vi "Read Write Config.vi"(0 "Config File":path, 2 "Read?":bool, 7 "Cluster In":T2, 11 "Error In":errorcluster) -> (8 "Cluster Out":T2, 15 "Error Out":errorcluster)   [LabVIEW 2013]
uses:
  TypeDef/StandConfigCluster.ctl
  <vilib>/Utility/config.llb/Write Key (String).vi
  <vilib>/Utility/config.llb/Write Key (Double).vi
  <vilib>/Utility/config.llb/Write Key (I32).vi
  <vilib>/Utility/config.llb/Read Key (String).vi
  <vilib>/Utility/config.llb/Read Key (Double).vi
  <vilib>/Utility/config.llb/Read Key (I32).vi
  <vilib>/Utility/config.llb/NI_LVConfig.lvlib
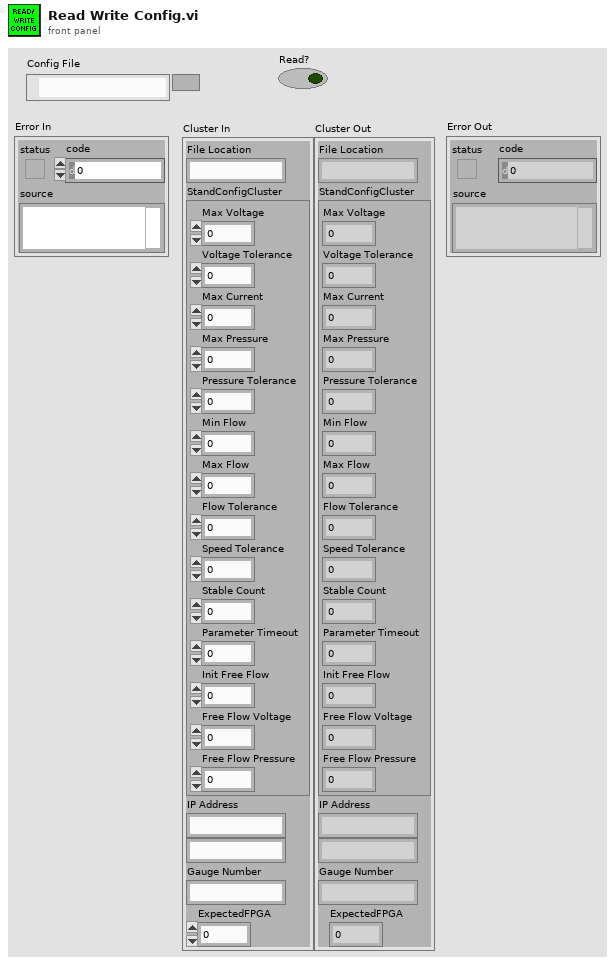
[diagram p1: front panel]
types:
  T1 = typedef "StandConfigCluster.ctl" = cluster{"Max Voltage":dbl, "Voltage Tolerance":dbl, "Max Current":dbl, "Max Pressure":dbl, "Pressure Tolerance":dbl, "Min Flow":dbl, "Max Flow":dbl, "Flow Tolerance":dbl, "Speed Tolerance":dbl, "Stable Count":dbl, "Parameter Timeout":dbl, "Init Free Flow":dbl, "Free Flow Voltage":dbl, "Free Flow Pressure":dbl}
  T2 = cluster{"File Location":string, "StandConfigCluster":T1, "IP Address":string, string, "Gauge Number":string, "ExpectedFPGA":i32}
  T3 = enum16{"open", "replace", "create", "open or create", "replace or create", "replace or create with confirmation"}
  T4 = typedef "NI_LVConfig.lvlib/Config Data RefNum.ctl" = refnum<k1>
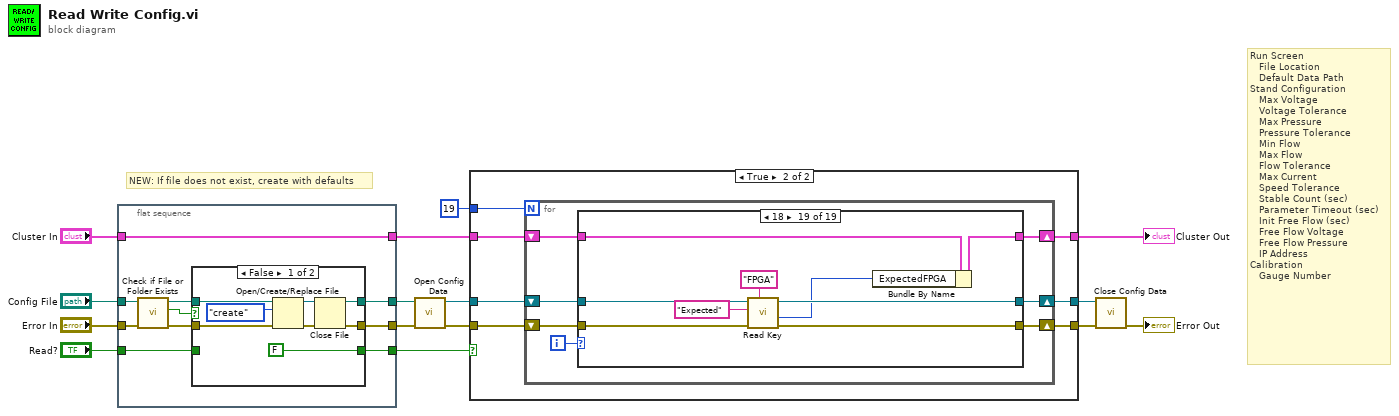
[diagram p0: block diagram]
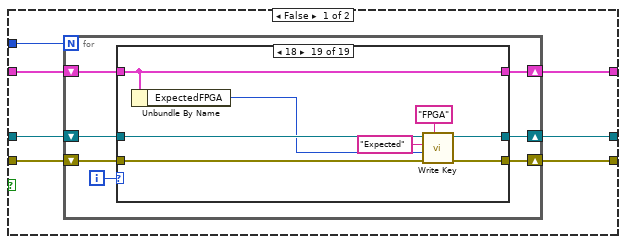
[diagram p3: hidden frame]
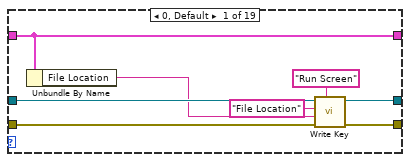
[diagram p4: hidden frame]
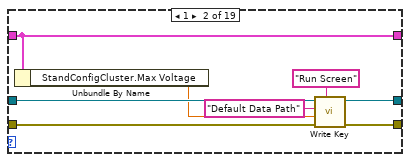
[diagram p5: hidden frame]
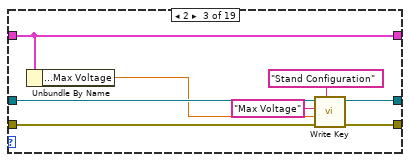
[diagram p6: hidden frame]
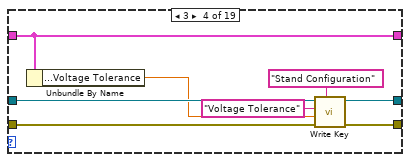
[diagram p7: hidden frame]
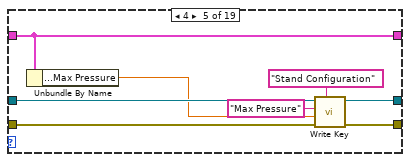
[diagram p8: hidden frame]
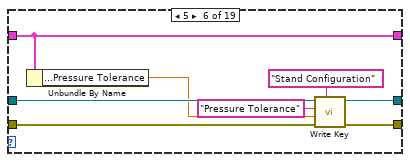
[diagram p9: hidden frame]
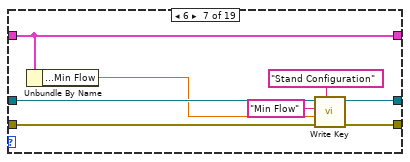
[diagram p10: hidden frame]
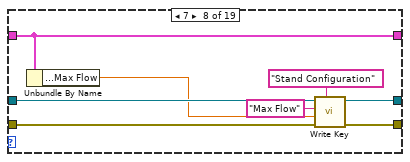
[diagram p11: hidden frame]
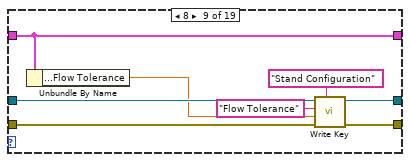
[diagram p12: hidden frame]
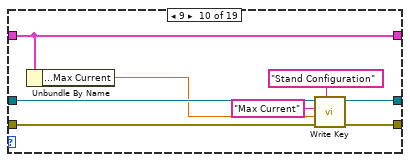
[diagram p13: hidden frame]
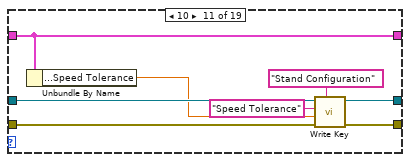
[diagram p14: hidden frame]
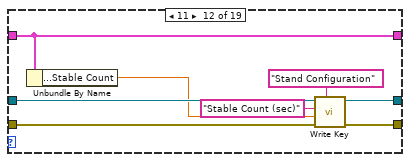
[diagram p15: hidden frame]
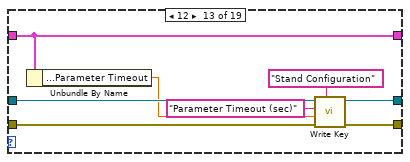
[diagram p16: hidden frame]
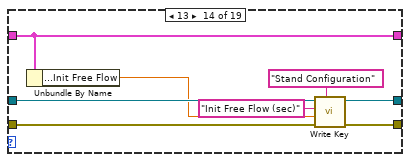
[diagram p17: hidden frame]
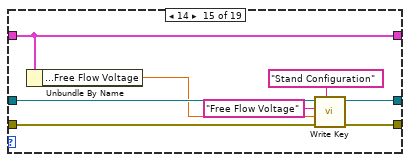
[diagram p18: hidden frame]
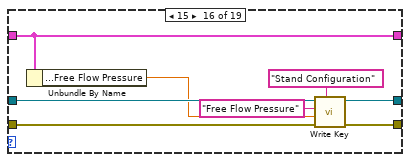
[diagram p19: hidden frame]
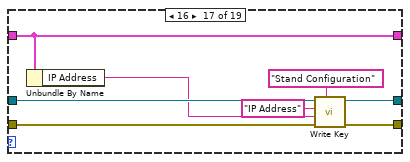
[diagram p20: hidden frame]
diagram:
  # "NEW: If file does not exist, create with defaults"
  # "Run Screen\n   File Location\n   Default Data Path\nStand Configuration\n   Max Voltage\n   Voltage Tolerance\n   Max Pressure\n   Pressure Tolerance\n   Min Flow\n   Max Flow\n   Flow Tolerance\n   Max Current\n   Speed Tolerance\n   Stable Count (sec)\n   Parameter Timeout (sec)\n   Init Free Flow (sec)\n   Free Flow Voltage\n   Free Flow Pressure\n   IP Address\nCalibration\n   Gauge Number"
  n1 = flat-sequence {
    tunnel: "Cluster In" -> [w25]
    tunnel: "Config File" -> [w24]
    tunnel: "Error In" -> [w23]
    tunnel: "Read?" -> [w17]
    tunnel: [w25] -> w7
    tunnel: [w19] -> w6
    tunnel: [w18] -> w5
    tunnel: [w16] -> w4
    frame #0 {
      n2 = call <vilib>:"Check if File or Folder Exists.vi"("error in (no error)"=w23, "path"=w24) -> ("error out"=w21:errorcluster, "file or folder exists?"=w22:bool, "dup path"=w20:path)  [unwired: 7 in]
      n3 = case shown="False" w22 {
        tunnel: [w28 w36] -> w18
        tunnel: w21 -> [w31 w36]
        tunnel: [w27 w35] -> w19
        tunnel: w20 -> [w32 w35]
        tunnel: [FALSE w34] -> w16
        tunnel: w17 -> [_ w34]
        frame False {
          n4 = Open/Create/Replace File(file path (use dialog)=w32, error in=w31, operation (0:open)=T3."create") -> (refnum out=w26:refnum<file>, error out=w29:errorcluster)  [unwired: 3 in, 1 out]
          n5 = Close File(refnum=w26, error in=w29) -> (path=w27:path, error out=w28:errorcluster)
        }
        frame True {
        }
      }
    }
  }
  n6 = call <vilib>:"Open Config Data.vi"("error in (no error)"=w5, "configuration file path"=w6) -> ("error out"=w14:errorcluster, "refnum"=w15:T4)  [unwired: 7 in, 1 out]
  n7 = case shown="True" w4 {
    tunnel: w15 -> [w43 w209]
    tunnel: w14 -> [w42 w208]
    tunnel: [w41 w207] -> w13
    tunnel: [w40 w206] -> w12
    tunnel: w7 -> [w39 w205]
    tunnel: [w38 w204] -> w1
    tunnel: 19 -> [w37 w203]
    frame False {
      n8 = for {
        N: w37 -> [_]
        shift-right: [w48] -> w41
        shift-left: w43 -> [w50]
        shift-right: [w47] -> w40
        shift-left: w42 -> [w49]
        shift-right: [w44] -> w38
        shift-left: w39 -> [w45]
        i -> [w46]
        n9 = case shown="18" w46 {
          tunnel: w50 -> [w58 w66 w74 w82 w90 w98 w106 w114 w122 w130 w138 w146 w154 w162 w170 w178 w186 w194 w202]
          tunnel: w49 -> [w57 w65 w73 w81 w89 w97 w105 w113 w121 w129 w137 w145 w153 w161 w169 w177 w185 w193 w201]
          tunnel: [w56 w64 w72 w80 w88 w96 w104 w112 w120 w128 w136 w144 w152 w160 w168 w176 w184 w192 w200] -> w48
          tunnel: [w55 w63 w71 w79 w87 w95 w103 w111 w119 w127 w135 w143 w151 w159 w167 w175 w183 w191 w199] -> w47
          tunnel: w45 -> [w52 w60 w68 w76 w84 w92 w100 w108 w116 w124 w132 w140 w148 w156 w164 w172 w180 w189 w197]
          tunnel: [w52 w60 w68 w76 w84 w92 w100 w108 w116 w124 w132 w140 w148 w156 w164 w172 w180 w189 w197] -> w44
          frame 0, Default {
            n10 = Unbundle By Name(w52) -> ("File Location"=w51:string)
            n11 = call-poly <vilib>:"Write Key.vi"("section"="Run Screen", "error in (no error)"=w57, "value"=w51, "key"="File Location", "refnum"=w58) -> ("error out"=w55:errorcluster, "refnum out"=w56:T4)  [unwired: 4 in, 1 out]
          }
          frame 1 {
            n12 = Unbundle By Name(w60) -> ("StandConfigCluster.Max Voltage"=w59:dbl)
            n13 = call-poly <vilib>:"Write Key.vi"("section"="Run Screen", "error in (no error)"=w65, "value"=w59, "key"="Default Data Path", "refnum"=w66) -> ("error out"=w63:errorcluster, "refnum out"=w64:T4)  [unwired: 4 in, 1 out]
          }
          frame 2 {
            n14 = Unbundle By Name(w68) -> ("StandConfigCluster.Max Voltage"=w67:dbl)
            n15 = call-poly <vilib>:"Write Key.vi"("section"="Stand Configuration", "error in (no error)"=w73, "value"=w67, "key"="Max Voltage", "refnum"=w74) -> ("error out"=w71:errorcluster, "refnum out"=w72:T4)  [unwired: 4 in, 1 out]
          }
          frame 3 {
            n16 = Unbundle By Name(w76) -> ("StandConfigCluster.Voltage Tolerance"=w75:dbl)
            n17 = call-poly <vilib>:"Write Key.vi"("section"="Stand Configuration", "error in (no error)"=w81, "value"=w75, "key"="Voltage Tolerance", "refnum"=w82) -> ("error out"=w79:errorcluster, "refnum out"=w80:T4)  [unwired: 4 in, 1 out]
          }
          frame 4 {
            n18 = Unbundle By Name(w84) -> ("StandConfigCluster.Max Pressure"=w83:dbl)
            n19 = call-poly <vilib>:"Write Key.vi"("section"="Stand Configuration", "error in (no error)"=w89, "value"=w83, "key"="Max Pressure", "refnum"=w90) -> ("error out"=w87:errorcluster, "refnum out"=w88:T4)  [unwired: 4 in, 1 out]
          }
          frame 5 {
            n20 = Unbundle By Name(w92) -> ("StandConfigCluster.Pressure Tolerance"=w91:dbl)
            n21 = call-poly <vilib>:"Write Key.vi"("section"="Stand Configuration", "error in (no error)"=w97, "value"=w91, "key"="Pressure Tolerance", "refnum"=w98) -> ("error out"=w95:errorcluster, "refnum out"=w96:T4)  [unwired: 4 in, 1 out]
          }
          frame 6 {
            n22 = Unbundle By Name(w100) -> ("StandConfigCluster.Min Flow"=w99:dbl)
            n23 = call-poly <vilib>:"Write Key.vi"("section"="Stand Configuration", "error in (no error)"=w105, "value"=w99, "key"="Min Flow", "refnum"=w106) -> ("error out"=w103:errorcluster, "refnum out"=w104:T4)  [unwired: 4 in, 1 out]
          }
          frame 7 {
            n24 = Unbundle By Name(w108) -> ("StandConfigCluster.Max Flow"=w107:dbl)
            n25 = call-poly <vilib>:"Write Key.vi"("section"="Stand Configuration", "error in (no error)"=w113, "value"=w107, "key"="Max Flow", "refnum"=w114) -> ("error out"=w111:errorcluster, "refnum out"=w112:T4)  [unwired: 4 in, 1 out]
          }
          frame 8 {
            n26 = Unbundle By Name(w116) -> ("StandConfigCluster.Flow Tolerance"=w115:dbl)
            n27 = call-poly <vilib>:"Write Key.vi"("section"="Stand Configuration", "error in (no error)"=w121, "value"=w115, "key"="Flow Tolerance", "refnum"=w122) -> ("error out"=w119:errorcluster, "refnum out"=w120:T4)  [unwired: 4 in, 1 out]
          }
          frame 9 {
            n28 = Unbundle By Name(w124) -> ("StandConfigCluster.Max Current"=w123:dbl)
            n29 = call-poly <vilib>:"Write Key.vi"("section"="Stand Configuration", "error in (no error)"=w129, "value"=w123, "key"="Max Current", "refnum"=w130) -> ("error out"=w127:errorcluster, "refnum out"=w128:T4)  [unwired: 4 in, 1 out]
          }
          frame 10 {
            n30 = Unbundle By Name(w132) -> ("StandConfigCluster.Speed Tolerance"=w131:dbl)
            n31 = call-poly <vilib>:"Write Key.vi"("section"="Stand Configuration", "error in (no error)"=w137, "value"=w131, "key"="Speed Tolerance", "refnum"=w138) -> ("error out"=w135:errorcluster, "refnum out"=w136:T4)  [unwired: 4 in, 1 out]
          }
          frame 11 {
            n32 = Unbundle By Name(w140) -> ("StandConfigCluster.Stable Count"=w139:dbl)
            n33 = call-poly <vilib>:"Write Key.vi"("section"="Stand Configuration", "error in (no error)"=w145, "value"=w139, "key"="Stable Count (sec)", "refnum"=w146) -> ("error out"=w143:errorcluster, "refnum out"=w144:T4)  [unwired: 4 in, 1 out]
          }
          frame 12 {
            n34 = Unbundle By Name(w148) -> ("StandConfigCluster.Parameter Timeout"=w147:dbl)
            n35 = call-poly <vilib>:"Write Key.vi"("section"="Stand Configuration", "error in (no error)"=w153, "value"=w147, "key"="Parameter Timeout (sec)", "refnum"=w154) -> ("error out"=w151:errorcluster, "refnum out"=w152:T4)  [unwired: 4 in, 1 out]
          }
          frame 13 {
            n36 = Unbundle By Name(w156) -> ("StandConfigCluster.Init Free Flow"=w155:dbl)
            n37 = call-poly <vilib>:"Write Key.vi"("section"="Stand Configuration", "error in (no error)"=w161, "value"=w155, "key"="Init Free Flow (sec)", "refnum"=w162) -> ("error out"=w159:errorcluster, "refnum out"=w160:T4)  [unwired: 4 in, 1 out]
          }
          frame 14 {
            n38 = Unbundle By Name(w164) -> ("StandConfigCluster.Free Flow Voltage"=w163:dbl)
            n39 = call-poly <vilib>:"Write Key.vi"("section"="Stand Configuration", "error in (no error)"=w169, "value"=w163, "key"="Free Flow Voltage", "refnum"=w170) -> ("error out"=w167:errorcluster, "refnum out"=w168:T4)  [unwired: 4 in, 1 out]
          }
          frame 15 {
            n40 = Unbundle By Name(w172) -> ("StandConfigCluster.Free Flow Pressure"=w171:dbl)
            n41 = call-poly <vilib>:"Write Key.vi"("section"="Stand Configuration", "error in (no error)"=w177, "value"=w171, "key"="Free Flow Pressure", "refnum"=w178) -> ("error out"=w175:errorcluster, "refnum out"=w176:T4)  [unwired: 4 in, 1 out]
          }
          frame 16 {
            n42 = Unbundle By Name(w180) -> ("IP Address"=w179:string)
            n43 = call-poly <vilib>:"Write Key.vi"("section"="Stand Configuration", "error in (no error)"=w185, "value"=w179, "key"="IP Address", "refnum"=w186) -> ("error out"=w183:errorcluster, "refnum out"=w184:T4)  [unwired: 4 in, 1 out]
          }
          frame 17 {
            n44 = Unbundle By Name(w189) -> ("Gauge Number"=w187:string)
            n45 = call-poly <vilib>:"Write Key.vi"("section"="Calibration", "error in (no error)"=w193, "value"=w187, "key"="Gauge Number", "refnum"=w194) -> ("error out"=w191:errorcluster, "refnum out"=w192:T4)  [unwired: 4 in, 1 out]
          }
          frame 18 {
            n46 = Unbundle By Name(w197) -> ("ExpectedFPGA"=w195:i32)
            n47 = call-poly <vilib>:"Write Key.vi"("section"="FPGA", "error in (no error)"=w201, "value"=w195, "key"="Expected", "refnum"=w202) -> ("error out"=w199:errorcluster, "refnum out"=w200:T4)  [unwired: 4 in, 1 out]
          }
        }
      }
    }
    frame True {
      n48 = for {
        N: w203 -> [_]
        shift-right: [w214] -> w207
        shift-left: w209 -> [w216]
        shift-right: [w213] -> w206
        shift-left: w208 -> [w215]
        shift-right: [w210] -> w204
        shift-left: w205 -> [w211]
        i -> [w212]
        n49 = case shown="18" w212 {
          tunnel: w216 -> [w225 w234 w243 w252 w261 w270 w279 w288 w297 w306 w315 w324 w333 w342 w351 w360 w369 w378 w387]
          tunnel: w215 -> [w224 w233 w242 w251 w260 w269 w278 w287 w296 w305 w314 w323 w332 w341 w350 w359 w368 w377 w386]
          tunnel: [w223 w232 w241 w250 w259 w268 w277 w286 w295 w304 w313 w322 w331 w340 w349 w358 w367 w376 w385] -> w214
          tunnel: [w222 w231 w240 w249 w258 w267 w276 w285 w294 w303 w312 w321 w330 w339 w348 w357 w366 w375 w384] -> w213
          tunnel: w211 -> [w221 w230 w239 w248 w257 w266 w275 w284 w293 w302 w311 w320 w329 w338 w347 w356 w365 w372 w381]
          tunnel: [w220 w229 w238 w247 w256 w265 w274 w283 w292 w301 w310 w319 w328 w337 w346 w355 w364 w371 w380] -> w210
          frame 0, Default {
            n50 = call-poly <vilib>:"Read Key.vi"("section"="Run Screen", "error in (no error)"=w224, "key"="File Location", "refnum"=w225) -> ("error out"=w222:errorcluster, "value"=w217:string, "refnum out"=w223:T4)  [unwired: 4 in, 1 out]
            n51 = Bundle By Name(cluster=w221, "File Location"=w217) -> (w220:T2)
          }
          frame 1 {
            n52 = call-poly <vilib>:"Read Key.vi"("section"="Run Screen", "error in (no error)"=w233, "key"="Default Data Path", "refnum"=w234) -> ("error out"=w231:errorcluster, "value"=w226:string, "refnum out"=w232:T4)  [unwired: 4 in, 1 out]
            n53 = Bundle By Name(cluster=w230, "File Location"=w226) -> (w229:T2)
          }
          frame 2 {
            n54 = call-poly <vilib>:"Read Key.vi"("section"="Stand Configuration", "error in (no error)"=w242, "key"="Max Voltage", "refnum"=w243) -> ("error out"=w240:errorcluster, "value"=w235:dbl, "refnum out"=w241:T4)  [unwired: 4 in, 1 out]
            n55 = Bundle By Name(cluster=w239, "StandConfigCluster.Max Voltage"=w235) -> (w238:T2)
          }
          frame 3 {
            n56 = call-poly <vilib>:"Read Key.vi"("section"="Stand Configuration", "error in (no error)"=w251, "key"="Voltage Tolerance", "refnum"=w252) -> ("error out"=w249:errorcluster, "value"=w244:dbl, "refnum out"=w250:T4)  [unwired: 4 in, 1 out]
            n57 = Bundle By Name(cluster=w248, "StandConfigCluster.Voltage Tolerance"=w244) -> (w247:T2)
          }
          frame 4 {
            n58 = call-poly <vilib>:"Read Key.vi"("section"="Stand Configuration", "error in (no error)"=w260, "key"="Max Pressure", "refnum"=w261) -> ("error out"=w258:errorcluster, "value"=w253:dbl, "refnum out"=w259:T4)  [unwired: 4 in, 1 out]
            n59 = Bundle By Name(cluster=w257, "StandConfigCluster.Max Pressure"=w253) -> (w256:T2)
          }
          frame 5 {
            n60 = call-poly <vilib>:"Read Key.vi"("section"="Stand Configuration", "error in (no error)"=w269, "key"="Pressure Tolerance", "refnum"=w270) -> ("error out"=w267:errorcluster, "value"=w262:dbl, "refnum out"=w268:T4)  [unwired: 4 in, 1 out]
            n61 = Bundle By Name(cluster=w266, "StandConfigCluster.Pressure Tolerance"=w262) -> (w265:T2)
          }
          frame 6 {
            n62 = call-poly <vilib>:"Read Key.vi"("section"="Stand Configuration", "error in (no error)"=w278, "key"="Min Flow", "refnum"=w279) -> ("error out"=w276:errorcluster, "value"=w271:dbl, "refnum out"=w277:T4)  [unwired: 4 in, 1 out]
            n63 = Bundle By Name(cluster=w275, "StandConfigCluster.Min Flow"=w271) -> (w274:T2)
          }
          frame 7 {
            n64 = call-poly <vilib>:"Read Key.vi"("section"="Stand Configuration", "error in (no error)"=w287, "key"="Max Flow", "refnum"=w288) -> ("error out"=w285:errorcluster, "value"=w280:dbl, "refnum out"=w286:T4)  [unwired: 4 in, 1 out]
            n65 = Bundle By Name(cluster=w284, "StandConfigCluster.Max Flow"=w280) -> (w283:T2)
          }
          frame 8 {
            n66 = call-poly <vilib>:"Read Key.vi"("section"="Stand Configuration", "error in (no error)"=w296, "key"="Flow Tolerance", "refnum"=w297) -> ("error out"=w294:errorcluster, "value"=w289:dbl, "refnum out"=w295:T4)  [unwired: 4 in, 1 out]
            n67 = Bundle By Name(cluster=w293, "StandConfigCluster.Flow Tolerance"=w289) -> (w292:T2)
          }
          frame 9 {
            n68 = call-poly <vilib>:"Read Key.vi"("section"="Stand Configuration", "error in (no error)"=w305, "key"="Max Current", "refnum"=w306) -> ("error out"=w303:errorcluster, "value"=w298:dbl, "refnum out"=w304:T4)  [unwired: 4 in, 1 out]
            n69 = Bundle By Name(cluster=w302, "StandConfigCluster.Max Current"=w298) -> (w301:T2)
          }
          frame 10 {
            n70 = call-poly <vilib>:"Read Key.vi"("section"="Stand Configuration", "error in (no error)"=w314, "key"="Speed Tolerance", "refnum"=w315) -> ("error out"=w312:errorcluster, "value"=w307:dbl, "refnum out"=w313:T4)  [unwired: 4 in, 1 out]
            n71 = Bundle By Name(cluster=w311, "StandConfigCluster.Speed Tolerance"=w307) -> (w310:T2)
          }
          frame 11 {
            n72 = call-poly <vilib>:"Read Key.vi"("section"="Stand Configuration", "error in (no error)"=w323, "key"="Stable Count (sec)", "refnum"=w324) -> ("error out"=w321:errorcluster, "value"=w316:dbl, "refnum out"=w322:T4)  [unwired: 4 in, 1 out]
            n73 = Bundle By Name(cluster=w320, "StandConfigCluster.Stable Count"=w316) -> (w319:T2)
          }
          frame 12 {
            n74 = call-poly <vilib>:"Read Key.vi"("section"="Stand Configuration", "error in (no error)"=w332, "key"="Parameter Timeout (sec)", "refnum"=w333) -> ("error out"=w330:errorcluster, "value"=w325:dbl, "refnum out"=w331:T4)  [unwired: 4 in, 1 out]
            n75 = Bundle By Name(cluster=w329, "StandConfigCluster.Parameter Timeout"=w325) -> (w328:T2)
          }
          frame 13 {
            n76 = call-poly <vilib>:"Read Key.vi"("section"="Stand Configuration", "error in (no error)"=w341, "key"="Init Free Flow (sec)", "refnum"=w342) -> ("error out"=w339:errorcluster, "value"=w334:dbl, "refnum out"=w340:T4)  [unwired: 4 in, 1 out]
            n77 = Bundle By Name(cluster=w338, "StandConfigCluster.Init Free Flow"=w334) -> (w337:T2)
          }
          frame 14 {
            n78 = call-poly <vilib>:"Read Key.vi"("section"="Stand Configuration", "error in (no error)"=w350, "key"="Free Flow Voltage", "refnum"=w351) -> ("error out"=w348:errorcluster, "value"=w343:dbl, "refnum out"=w349:T4)  [unwired: 4 in, 1 out]
            n79 = Bundle By Name(cluster=w347, "StandConfigCluster.Free Flow Voltage"=w343) -> (w346:T2)
          }
          frame 15 {
            n80 = call-poly <vilib>:"Read Key.vi"("section"="Stand Configuration", "error in (no error)"=w359, "key"="Free Flow Pressure", "refnum"=w360) -> ("error out"=w357:errorcluster, "value"=w352:dbl, "refnum out"=w358:T4)  [unwired: 4 in, 1 out]
            n81 = Bundle By Name(cluster=w356, "StandConfigCluster.Free Flow Pressure"=w352) -> (w355:T2)
          }
          frame 16 {
            n82 = call-poly <vilib>:"Read Key.vi"("section"="Stand Configuration", "error in (no error)"=w368, "key"="IP Address", "refnum"=w369) -> ("error out"=w366:errorcluster, "value"=w361:string, "refnum out"=w367:T4)  [unwired: 4 in, 1 out]
            n83 = Bundle By Name(cluster=w365, "IP Address"=w361) -> (w364:T2)
          }
          frame 17 {
            n84 = call-poly <vilib>:"Read Key.vi"("section"="Calibration", "error in (no error)"=w377, "key"="Gauge Number", "refnum"=w378) -> ("error out"=w375:errorcluster, "value"=w370:string, "refnum out"=w376:T4)  [unwired: 4 in, 1 out]
            n85 = Bundle By Name(cluster=w372, "Gauge Number"=w370) -> (w371:T2)
          }
          frame 18 {
            n86 = call-poly <vilib>:"Read Key.vi"("section"="FPGA", "error in (no error)"=w386, "key"="Expected", "refnum"=w387) -> ("error out"=w384:errorcluster, "value"=w379:i32, "refnum out"=w385:T4)  [unwired: 4 in, 1 out]
            n87 = Bundle By Name(cluster=w381, "ExpectedFPGA"=w379) -> (w380:T2)
          }
        }
      }
    }
  }
  "Cluster Out" <- w1
  n88 = call <vilib>:"Close Config Data.vi"("error in (no error)"=w12, "refnum"=w13) -> ("error out"=→"Error Out":errorcluster)  [unwired: 8 in, 1 out]
